vi "Build core.vi"(6 "Previous Build's Artifacts":refnum<class "Build Artifact.lvclass">[](array[class]), 7 "Progress":refnum<class "Progress.lvclass">, 8 "error in (no error)":errorcluster, 10 "Build Cache":refnum<class "Build Cache.lvclass">, 11 "Open VIPM Step in":refnum<class "Open VIPM Step.lvclass">) -> (0 "error out":errorcluster, 1 "Explore Path":path, 2 "Build Results":T1, 4 "New Artifacts":refnum<class "Build Artifact.lvclass">[](array[class]))   [LabVIEW 2019, in "VIPM.lvlib" / "Open VIPM Step.lvclass"]
doc: "Performs all the necessary build actions for the build step.\n\nCopyright: MGI 2016\nAuthor: Derek Trepanier"
uses:
  Open VIPM Step.lvclass
  libs/Solution.lvlibp/Solution/Progress/Progress.lvclass
  libs/Solution.lvlibp/Solution/Build Artifact/Build Artifact.lvclass
  libs/Solution.lvlibp/Solution/Build Item/Build Result.ctl
  libs/Solution.lvlibp/Solution/Build Cache/Build Cache.lvclass
  <vilib>/JKI/VIPM API/VIPM API_vipm_api.lvlib
  libs/Solution.lvlibp/Solution/Build Item/Build Step.lvclass
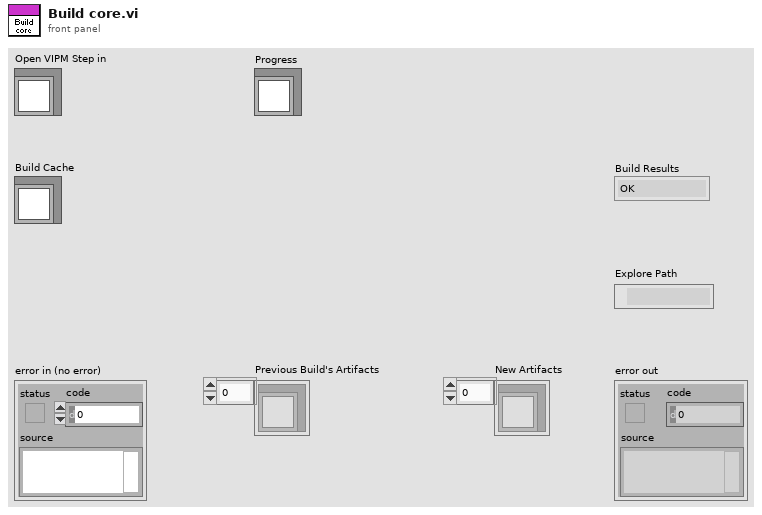
[diagram p1: front panel]
types:
  T1 = typedef "Solution.lvlibp/Build Step.lvclass/Build Result.ctl" = enum16{"OK", "Skipped", "Error"}
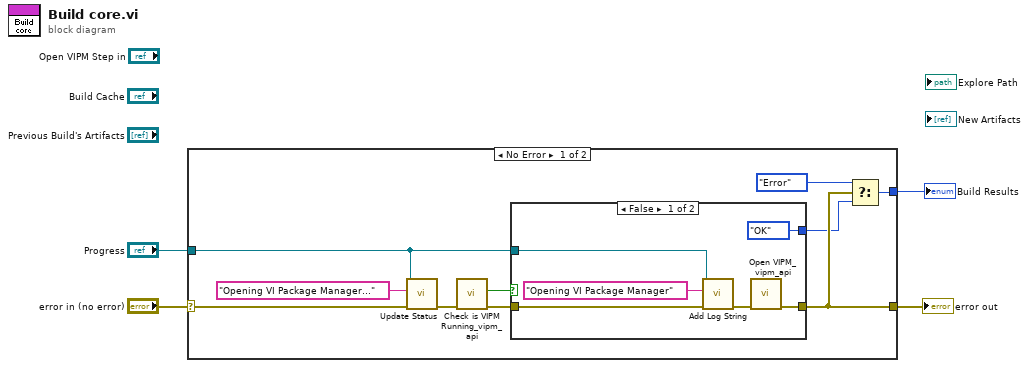
[diagram p0: block diagram]
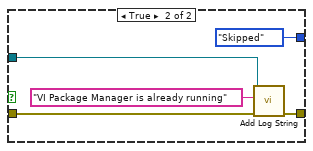
[diagram p2: hidden frame]
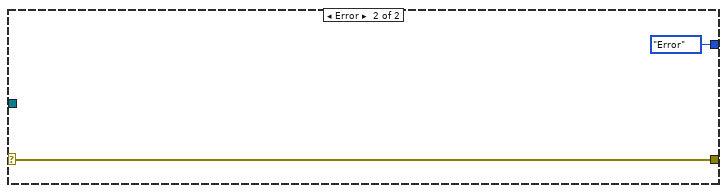
[diagram p3: hidden frame]
diagram:
  n1 = case shown="No Error" "error in (no error)" {
    selector: "error in (no error)" -> [w13 w26]
    tunnel: "Progress" -> [w11 _]
    tunnel: [w10 Build_Result."Error" ("Build Results")] -> w2
    tunnel: [w9 w26] -> w1
    frame No Error {
      n2 = call "Update Status.vi"("error in (no error)"=w13, "Status String"="Opening VI Package Manager...", "Progress in"=w11) -> ("error out"=w5:errorcluster)  [unwired: 8 in]
      n3 = call <vilib>:"Check is VIPM Running_vipm_api.vi"("error in (no error)"=w5) -> ("error out"=w14:errorcluster, "is Running"=w7:bool)  [unwired: 9 in]
      n4 = case shown="False" w7 {
        tunnel: [w20 w24] -> w9
        tunnel: w14 -> [w17 w25]
        tunnel: w11 -> [w16 w23]
        tunnel: [Build_Result."OK" ("Build Results") Build_Result."Skipped" ("Build Results")] -> w6
        frame False {
          n5 = call "Add Log String.vi"("error in (no error)"=w17, "Log Item"="Opening VI Package Manager", "Progress in"=w16) -> ("error out"=w18:errorcluster)  [unwired: 8 in]
          n6 = call <vilib>:"Open VIPM_vipm_api.vi"("error in (no error)"=w18) -> ("error out"=w20:errorcluster)  [unwired: 10 in]
        }
        frame True {
          n7 = call "Add Log String.vi"("error in (no error)"=w25, "Log Item"="VI Package Manager is already running", "Progress in"=w23) -> ("error out"=w24:errorcluster)  [unwired: 8 in]
        }
      }
      n8 = Select(t=Build_Result."Error" ("Build Results"), s=w9, f=w6) -> (s? t:f=w10:T1)
    }
    frame Error {
    }
  }
  "error out" <- w1
  "Build Results" <- w2
